vi "W vs Z main7b.vi"() -> ()   [LabVIEW 2012]
panel:
  in  "Lens 4 Params":T1={"Focal length"=0.0, "Index in"=1.0, " Index out"=1.0} {"Index out" format="%.2f"; "Index in" format="%.2f"; "Focal length" format="%.2f"}
  in  "Lens 3 Params":T1={"Focal length"=0.0, "Index in"=1.0, " Index out"=1.0} {"Index out" format="%.2f"; "Index in" format="%.2f"; "Focal length" format="%.2f"}
  in  "Lens 2 Params":T1={"Focal length"=0.0, "Index in"=1.0, " Index out"=1.0} {"Index out" format="%.2f"; "Index in" format="%.2f"; "Focal length" format="%.2f"}
  in  "Lens 1 Params":T1={"Focal length"=0.0, "Index in"=1.0, " Index out"=1.0} {"Index out" format="%.2f"; "Index in" format="%.2f"; "Focal length" format="%.2f"}
  out "lens 4 position":dbl
  out "lens 1-2 separation":dbl
  in  "FWHM(T)?":bool
  out "contains waist? 1":bool
  out "contains waist? 3":bool
  out "contains waist? 2":bool
  out "FWHM1":dbl format="%.5f"
  out "FWHM3":dbl format="%.5f"
  out "FWHM2":dbl format="%.5f"
  out "Cursor List":T2(array[cluster]) {"Location"."Y" format="%.2f"; "Location"."X" format="%.2f"}
  out "Zor FWHM Array 3":dbl[](array[numeric]) format="%.2f"
  out "Z Array 2":dbl[](array[numeric]) format="%.2f"
  out "Z Array":dbl[](array[numeric]) format="%.2f"
  out "w Array 3":dbl[](array[numeric]) format="%.2f"
  out "w Array 2":dbl[](array[numeric]) format="%.2f"
  out "w Array":dbl[](array[numeric]) format="%.2f"
  out "min w 1":dbl format="%.5f"
  out "min w 3":dbl format="%.5f"
  in  "z stop":dbl=1000.0 format="%.2f"
  in  "N steps":i32=500
  out "min  z 2":dbl format="%.2f"
  out "min z 1":dbl format="%.2f"
  out "min Z 3":dbl format="%.2f"
  out "min w 2":dbl format="%.5f"
  out "Q start":cdb format="%.4f"
  out "W vs Z":cluster{dbl[], dbl[]}[](graph)
  in  "beam radius(w)":dbl=0.6 format="%.4f"
  in  "Radius of Curvature":dbl=inf format="%.2f"
  in  "Wavelength":dbl=0.00035 format="%.6f"
  in  "z start":dbl format="%.2f"
  # "This version allows the lenses to be used as an index interface\ni.e. going from one media index to another\nA flat surface would have the f set to Inf and the in and out indexes\nset to not 1"
  # "All values are entered in mm"
  # "w is the 1/e field radius"
  # "w x 1.18 to get FWHM of the Intensity"
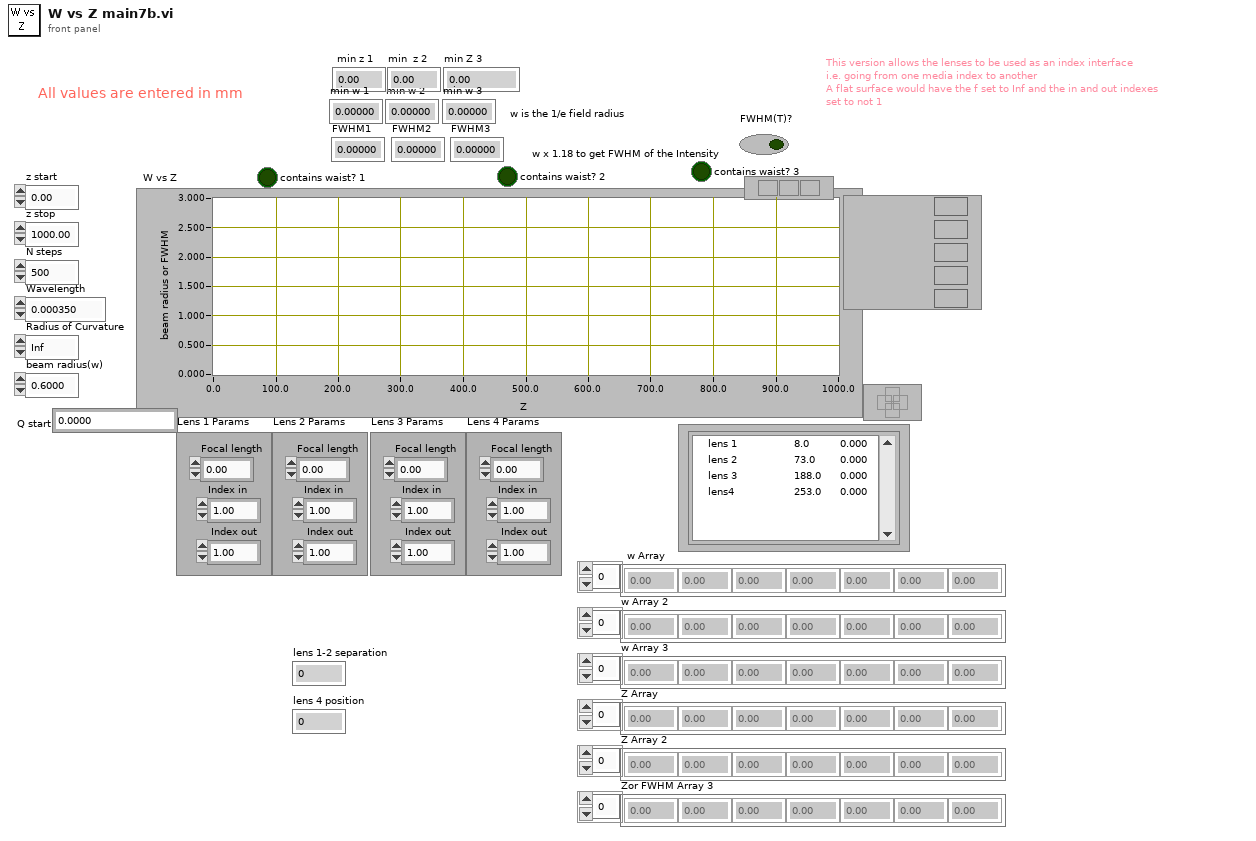
[diagram p1: front panel]
types:
  T1 = cluster{"Focal length":dbl, "Index in":dbl, " Index out":dbl}
  T2 = cluster{"Name":string, "Color":u32, "Hair Style":u8, "Point Style":u8, "Name Visible":bool, "Trackable":bool, "Lock Style":u32, "Plot Number":u32, "Marker Index":i32, "Location":cluster{"X":dbl, "Y":dbl}}[]
  T3 = cluster{"Name":string, "Color":u32, "Style":u8, "Point Style":u8, "Name Visible":bool, "Allow Drag":bool, "Lock Style":u32, "Plot":u32, "Index":i32, "Position":cluster{"X":dbl, "Y":dbl}}[]
  T4 = cluster{"Name":string, "Color":u32, "Style":u8, "Point Style":u8, "Name Visible":bool, "Allow Drag":bool, "Lock Style":u32, "Plot":u32, "Index":i32, "Position":cluster{"X":dbl, "Y":dbl}}
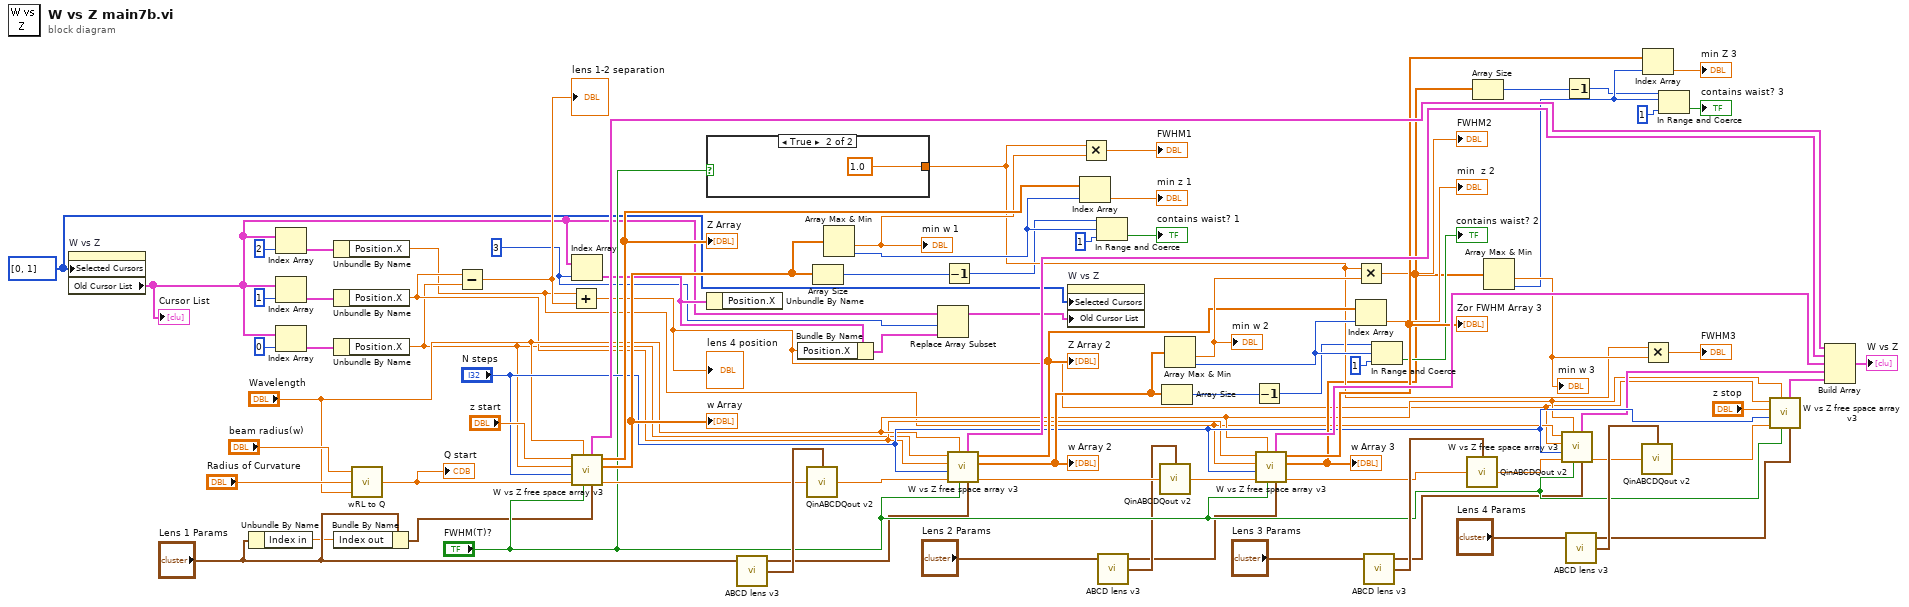
[diagram p0: block diagram]
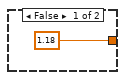
[diagram p2: hidden frame]
diagram:
  w15 = 3 ("Index")
  w14 = u32[] [0, 1] ("Selected Cursors")
  n1 = property on="W vs Z" class="XYGraph (strict)"("Selected Cursors"=w14) -> ("Old Cursor List"=w17:T3)  [unwired: 2 in, 2 out]
  "Cursor List" <- w17
  n2 = Unbundle By Name("Lens 1 Params") -> ("Index in"=w2:dbl)
  n3 = Index Array(array=w17, index=2 ("Index")) -> (element=w28:T4)
  n4 = Index Array(array=w17, index=1 ("Index")) -> (element=w69:T4)
  n5 = Index Array(array=w17, index=0 ("Index")) -> (element=w71:T4)
  n6 = Unbundle By Name(w28) -> ("Position.X"=w20:dbl)
  n7 = Unbundle By Name(w69) -> ("Position.X"=w23:dbl)
  n8 = Unbundle By Name(w71) -> ("Position.X"=w22:dbl)
  n9 = Bundle By Name(cluster="Lens 1 Params", "Index out"=w2) -> (w1:T1)
  n10 = call "wRL to Q.vi"("Wavelength"="Wavelength", "Radius of Curvature"="Radius of Curvature", "beam radius(w)"="beam radius(w)") -> ("Q"=w80:cdb)
  "Q start" <- w80
  n11 = Subtract(x=w23, y=w22) -> (x-y=w21:dbl)
  "lens 1-2 separation" <- w21
  n12 = Add(x=w20, y=w21) -> (x+y=w18:dbl)
  "lens 4 position" <- w18
  n13 = Index Array(array=w17, index=w15) -> (element=w19:T4)
  n14 = call "W vs Z free space array v3.vi"("Lens Params"=w1, "FWHM(T)?"="FWHM(T)?", "Wavelength"="Wavelength", "Q start"=w80, "N steps"="N steps", "z stop"=w22, "z start"="z start") -> ("Q out"=w78:cdb, "w/FWHM Array"=w39:dbl[], "Z Array"=w67:dbl[], "W/FWHM vs Z"=w76:cluster{dbl[], dbl[]})  [unwired: 1 out]
  "w Array" <- w39
  "Z Array" <- w67
  n15 = case shown="True" "FWHM(T)?" {
    tunnel: [1.18 ("x") 1.0 ("x")] -> w53
    frame False {
    }
    frame True {
    }
  }
  n16 = Unbundle By Name(w19) -> ()  [unwired: 1 out]
  n17 = call "ABCD lens v3.vi"("Lens Params"="Lens 1 Params") -> ("ABCD"=w82:cluster{"A":dbl, "B":dbl, "C":dbl, "D":dbl}, "Lens Params out"=w4:T1)  [unwired: 3 out]
  n18 = Bundle By Name(cluster=w19, "Position.X"=w18) -> (w16:T4)
  n19 = call "QinABCDQout v2.vi"("Q in"=w78, "ABCD"=w82) -> ("Q out"=w81:cdb)
  n20 = Array Size(array=w39) -> (size(s)=w44:i32)
  n21 = Array Max & Min(array=w39) -> (min value=w56:dbl, min index (indices)=w66:i32)  [unwired: 2 out]
  "min w 1" <- w56
  n22 = Replace Array Subset(array=w17, new element=w16, index=w15) -> (w13:T3)
  n23 = Decrement(x=w44) -> (x-1=w42:i32)
  n24 = call "W vs Z free space array v3.vi"("Lens Params"=w4, "FWHM(T)?"="FWHM(T)?", "Wavelength"="Wavelength", "Q start"=w81, "N steps"="N steps", "z stop"=w23, "z start"=w22) -> ("Q out"=w12:cdb, "w/FWHM Array"=w52:dbl[], "Z Array"=w62:dbl[], "W/FWHM vs Z"=w75:cluster{dbl[], dbl[]})  [unwired: 1 out]
  "w Array 2" <- w52
  "Z Array 2" <- w62
  n25 = property on="W vs Z" class="XYGraph (strict)"("Selected Cursors"=w14, "Old Cursor List"=w13) -> ()  [unwired: 2 in, 2 out]
  n26 = Index Array(array=w67, index=w66) -> (element=→"min z 1":dbl)
  n27 = Multiply(x=w53, y=w56) -> (x*y=→"FWHM1":dbl)
  n28 = In Range and Coerce(upper limit=w42, x=w66, lower limit=1) -> (In Range?=→"contains waist? 1":bool)  [unwired: 1 out]
  n29 = call "ABCD lens v3.vi"("Lens Params"="Lens 2 Params") -> ("ABCD"=w11:cluster{"A":dbl, "B":dbl, "C":dbl, "D":dbl}, "Lens Params out"=w6:T1)  [unwired: 3 out]
  n30 = call "QinABCDQout v2.vi"("Q in"=w12, "ABCD"=w11) -> ("Q out"=w77:cdb)
  n31 = Array Size(array=w52) -> (size(s)=w51:i32)
  n32 = Array Max & Min(array=w52) -> (min value=w64:dbl, min index (indices)=w63:i32)  [unwired: 2 out]
  "min w 2" <- w64
  n33 = Decrement(x=w51) -> (x-1=w48:i32)
  n34 = call "W vs Z free space array v3.vi"("Lens Params"=w6, "FWHM(T)?"="FWHM(T)?", "Wavelength"="Wavelength", "Q start"=w77, "N steps"="N steps", "z stop"=w20, "z start"=w23) -> ("Q out"=w32:cdb, "w/FWHM Array"=w41:dbl[], "Z Array"=w59:dbl[], "W/FWHM vs Z"=w74:cluster{dbl[], dbl[]})  [unwired: 1 out]
  "w Array 3" <- w41
  "Zor FWHM Array 3" <- w59
  n35 = Multiply(x=w53, y=w64) -> (x*y=→"FWHM2":dbl)
  n36 = Index Array(array=w62, index=w63) -> (element=→"min  z 2":dbl)
  n37 = call "ABCD lens v3.vi"("Lens Params"="Lens 3 Params") -> ("ABCD"=w37:cluster{"A":dbl, "B":dbl, "C":dbl, "D":dbl}, "Lens Params out"=w7:T1)  [unwired: 3 out]
  n38 = In Range and Coerce(upper limit=w48, x=w63, lower limit=1) -> (In Range?=→"contains waist? 2":bool)  [unwired: 1 out]
  n39 = call "QinABCDQout v2.vi"("Q in"=w32, "ABCD"=w37) -> ("Q out"=w36:cdb)
  n40 = Array Size(array=w41) -> (size(s)=w47:i32)
  n41 = Array Max & Min(array=w41) -> (min value=w73:dbl, min index (indices)=w60:i32)  [unwired: 2 out]
  "min w 3" <- w73
  n42 = call "W vs Z free space array v3.vi"("Lens Params"=w7, "FWHM(T)?"="FWHM(T)?", "Wavelength"="Wavelength", "Q start"=w36, "N steps"="N steps", "z stop"=w18, "z start"=w20) -> ("Q out"=w34:cdb, "W/FWHM vs Z"=w26:cluster{dbl[], dbl[]})  [unwired: 3 out]
  n43 = Decrement(x=w47) -> (x-1=w45:i32)
  n44 = call "ABCD lens v3.vi"("Lens Params"="Lens 4 Params") -> ("ABCD"=w35:cluster{"A":dbl, "B":dbl, "C":dbl, "D":dbl}, "Lens Params out"=w5:T1)  [unwired: 3 out]
  n45 = call "QinABCDQout v2.vi"("Q in"=w34, "ABCD"=w35) -> ("Q out"=w33:cdb)
  n46 = Index Array(array=w59, index=w60) -> (element=→"min Z 3":dbl)
  n47 = Multiply(x=w53, y=w73) -> (x*y=→"FWHM3":dbl)
  n48 = In Range and Coerce(upper limit=w45, x=w60, lower limit=1) -> (In Range?=→"contains waist? 3":bool)  [unwired: 1 out]
  n49 = call "W vs Z free space array v3.vi"("Lens Params"=w5, "FWHM(T)?"="FWHM(T)?", "Wavelength"="Wavelength", "Q start"=w33, "N steps"="N steps", "z stop"="z stop", "z start"=w18) -> ("W/FWHM vs Z"=w25:cluster{dbl[], dbl[]})  [unwired: 4 out]
  n50 = Build Array(w76, w75, w74, w26, w25) -> (→"W vs Z":cluster{dbl[], dbl[]}[])
